vi "Write.vi"(8 "error in (no error)":errorcluster, 9 "timeout (ms)":i32=1000, 10 "pcap L2Enet DATA in":u8[](array[numeric]), 11 "L2Enet_RW_CORE in":refnum<class "L2ENET_RW_CORE.lvclass">) -> (0 "error out":errorcluster, 3 "L2Enet_RW_CORE out":refnum<class "L2ENET_RW_CORE.lvclass">, 4 "number written":i32=-1)   [LabVIEW 2021, in "L2ENET_RW_CORE.lvclass"]
uses:
  L2ENET_RW_CORE.lvclass
  L2ENET_RW_CORE.lvclass/L2ENET_RW_CORE.ctl
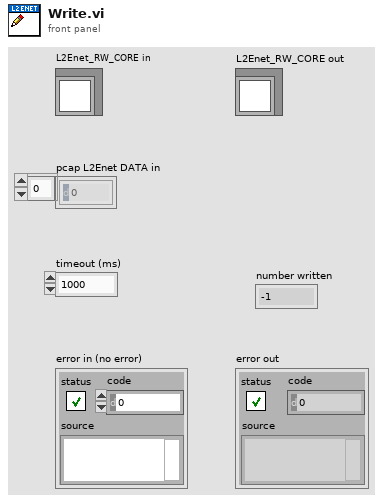
[diagram p1: front panel]
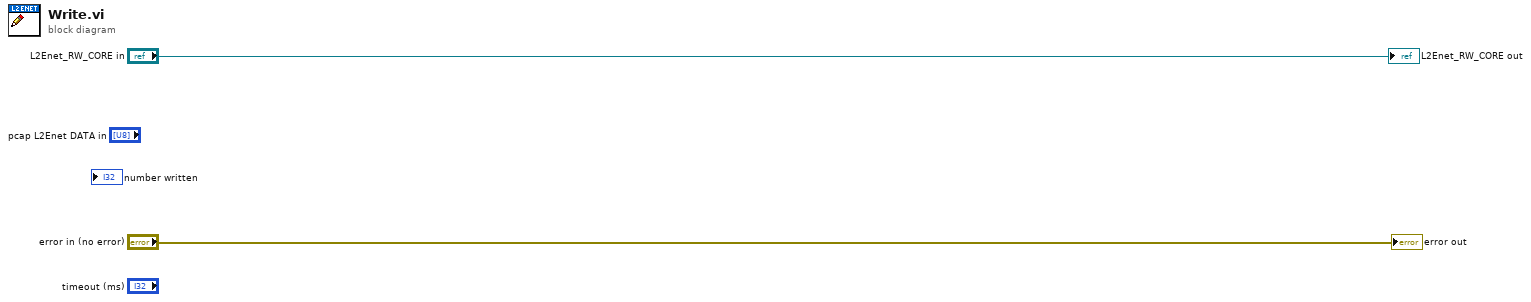
[diagram p0: block diagram]
diagram:
  "error out" <- "error in (no error)"
  "L2Enet_RW_CORE out" <- "L2Enet_RW_CORE in"
